vi "Connect.vi"(8 "error in (no error)":errorcluster, 11 "BASE.Device in":refnum<class "BASE.Device.lvclass">) -> (0 "error out":errorcluster, 3 "BASE.Device out":refnum<class "BASE.Device.lvclass">)   [LabVIEW 2019, in "BASE.Device.lvlib" / "BASE.Device.lvclass"]
uses:
  BASE.Device.lvclass
  BASE.Device.lvclass/BASE.Device.ctl
panel:
  in  "Blocking?":bool
  in  "Timeout (5000 ms)":i32
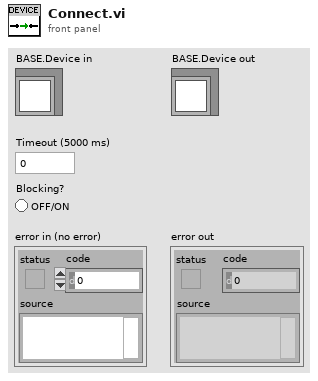
[diagram p1: front panel]
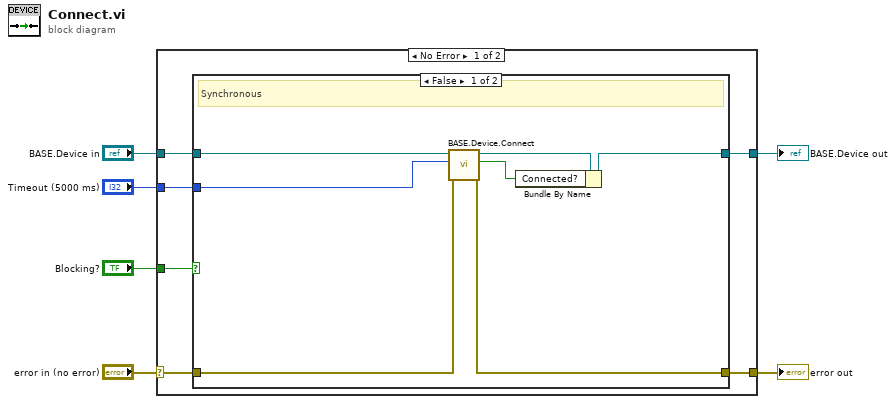
[diagram p0: block diagram]
diagram:
  n1 = case shown="No Error" "error in (no error)" {
    selector: "error in (no error)" -> [w12 w23]
    tunnel: [w11 w23] -> w5
    tunnel: [w9 w22] -> w3
    tunnel: "BASE.Device in" -> [w10 w22]
    tunnel: "Timeout (5000 ms)" -> [w8 _]
    tunnel: "Blocking?" -> [w7 _]
    frame No Error {
      n2 = case shown="False" w7 {
        tunnel: w8 -> [w13 _]
        tunnel: w10 -> [w18 w21]
        tunnel: [w19 w21] -> w9
        tunnel: w12 -> [w16 w20]
        tunnel: [w15 w20] -> w11
        frame False {
          # "Synchronous"
          n3 = call-dynamic "BASE.Device.Connect.vi"("error in (no error)"=w16, "Timeout (5000 ms)"=w13, "BASE.Device in"=w18) -> ("error out"=w15:errorcluster, "Connected?"=w14:bool, "BASE.Device out"=w17:refnum<class "BASE.Device.lvclass">)  [unwired: 6 in]
          n4 = Bundle By Name(cluster=w17, "Connected?"=w14) -> (w19:refnum<class "BASE.Device.lvclass">)
        }
        frame True {
          # "Aynchronous"
        }
      }
    }
    frame Error {
    }
  }
  "error out" <- w5
  "BASE.Device out" <- w3
